vi "Set_2G_RACH_Access_Control_Class.vi"(8 "error in (no error)":errorcluster, 10 "value":i32 min=0 max=16, 11 "Base Station":T1) -> (0 "error out":errorcluster, 3 "Output String":string)   [LabVIEW 2021]
uses:
  Controls/Base_Station_Emulator.ctl
  Controls/TCP_FGV.ctl
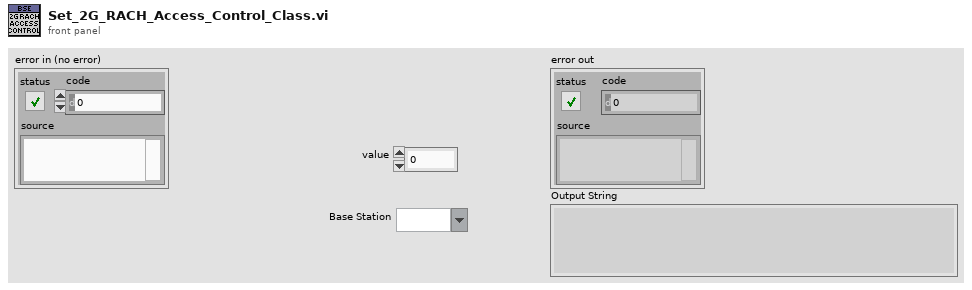
[diagram p1: front panel]
types:
  T1 = typedef "Base_Station_Emulator.ctl" = string
  T2 = typedef "TCP_FGV.ctl" = enum16{"Open", "Read", "Write", "Close"}
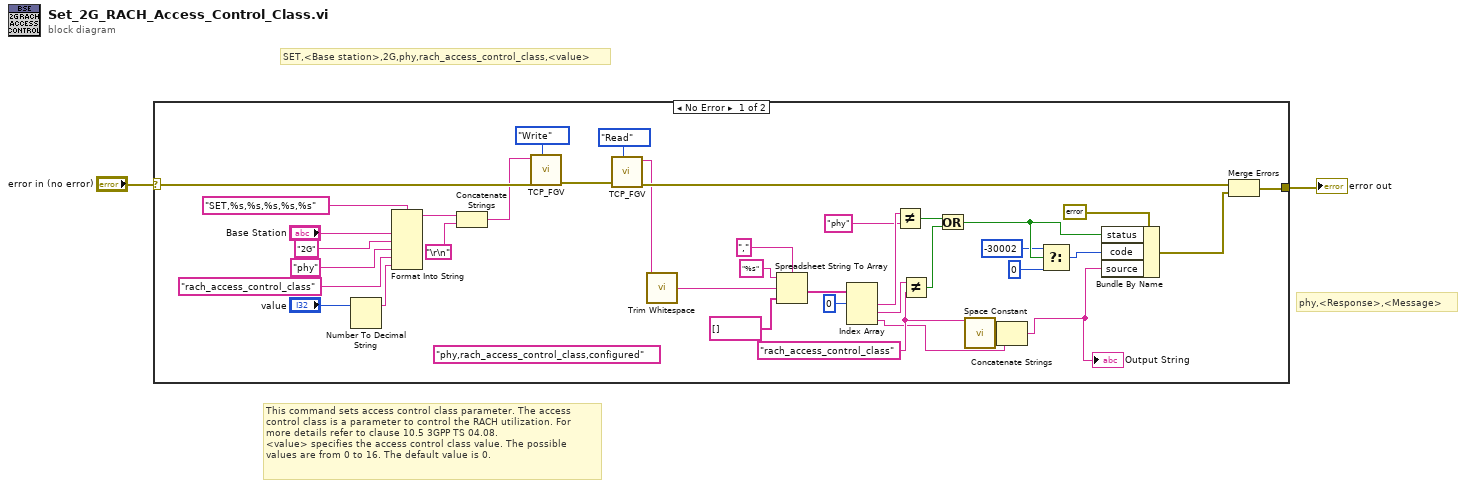
[diagram p0: block diagram]
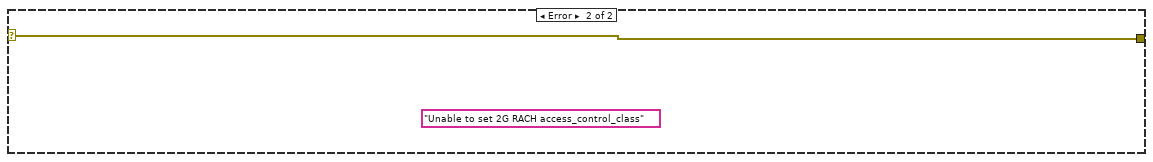
[diagram p2: hidden frame]
diagram:
  # "This command sets access control class parameter. The access \ncontrol class is a parameter to control the RACH utilization. For \nmore details refer to clause 10.5 3GPP TS 04.08.  \n<value> specifies the access control class value. The possible \nvalues are from 0 to 16. The default value is 0."
  # "phy,<Response>,<Message>"
  # "SET,<Base station>,2G,phy,rach_access_control_class,<value>"
  n1 = case shown="No Error" "error in (no error)" {
    selector: "error in (no error)" -> [w37 w41]
    tunnel: [w13 w41] -> w1
    frame No Error {
      (unwired) "phy,rach_access_control_class,configured" ("format string")
      w11 = "rach_access_control_class"
      n2 = Number To Decimal String(number="value") -> (decimal integer string=w6:string)  [unwired: 1 in]
      n3 = Format Into String(format string="SET,%s,%s,%s,%s,%s", "Base Station", "2G", "phy", "rach_access_control_class", w6) -> (resulting string=w4:string)  [unwired: 2 in, 1 out]
      n4 = Concatenate Strings(w4, "\r\n") -> (w3:string)
      n5 = call "TCP_FGV.vi"("Command"=w3, "error in (no error)"=w37, "Operation"=TCP_FGV."Write") -> ("error out"=w14:errorcluster)  [unwired: 6 in, 1 out]
      n6 = call "TCP_FGV.vi"("error in (no error)"=w14, "Operation"=TCP_FGV."Read") -> ("Data Out"=w15:string, "error out"=w17:errorcluster)  [unwired: 7 in]
      n7 = call <vilib>:"Trim Whitespace.vi"("string"=w15) -> ("trimmed string"=w31:string)  [unwired: 1 in]
      n8 = Spreadsheet String To Array(delimiter (Tab)=",", format string="%s", spreadsheet string=w31, array type (2D Dbl)=string[] []) -> (array=w27:string[])
      n9 = Index Array(array=w27, index #1=0 ("index")) -> (element #1=w28:string, element #2=w18:string, element #3=w10:string)  [unwired: 2 in]
      n10 = Not Equal?(x=w28, y="phy" ("format string")) -> (x != y?=w29:bool)
      n11 = Not Equal?(x=w18, y=w11) -> (x != y?=w30:bool)
      n12 = Or(x=w29, y=w30) -> (x .or. y?=w32:bool)
      n13 = call <vilib>:"Space Constant.vi"() -> ("String"=w12:string)
      n14 = Concatenate Strings(w11, w12, w10) -> (w9:string)
      "Output String" <- w9
      n15 = Select(t=-30002 ("code"), s=w32, f=0 ("code")) -> (s? t:f=w33:i32)
      n16 = Bundle By Name(cluster=errorcluster {"status"=FALSE, "code"=0, "source"=""} ("error constant"), "status"=w32, "code"=w33, "source"=w9) -> (w16:errorcluster)
      n17 = Merge Errors(w17, w16) -> (w13:errorcluster)
    }
    frame Error {
      (unwired) "Unable to set 2G RACH access_control_class" ("source")
    }
  }
  "error out" <- w1
